vi "Build Sensor Directory Path.vi"(11 "Top Level Path":path) -> (3 "Sensor Directory Path":path)   [LabVIEW 2013, in "File IO.lvlib"]
uses:
  File IO.lvlib
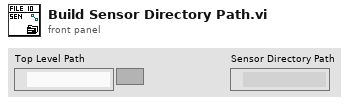
[diagram p1: front panel]
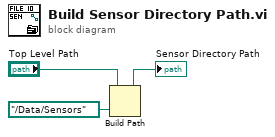
[diagram p0: block diagram]
diagram:
  n1 = Build Path(base path="Top Level Path", name or relative path=path "../Data/Sensors") -> (appended path=→"Sensor Directory Path":path)
